vi "Utility Write To Register.vi"(7 "Unit Address (1)":u8=1, 8 "error in (no error)":errorcluster, 9 "Data (0)":i16, 10 "Register Address (0)":u16, 11 "VISA resource name":refnum<visa-resource-name>) -> (0 "error out":errorcluster {"code" format="%.0x"}, 3 "VISA resource name out":refnum<visa-resource-name>)   [LabVIEW 2014, in "Eurotherm 35xx Series.lvlib"]
doc: "This VI writes the value to the specified register of specified unit."
uses:
  <instrlib>/Eurotherm 35xx Series/Eurotherm 35xx Series.lvlib
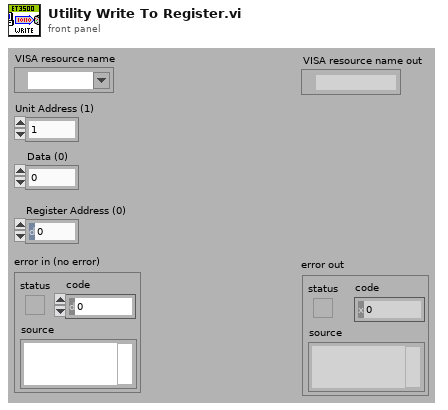
[diagram p1: front panel]
types:
  T1 = enum16{"By The Number of Bytes", "Copy Of the Sent Message"}
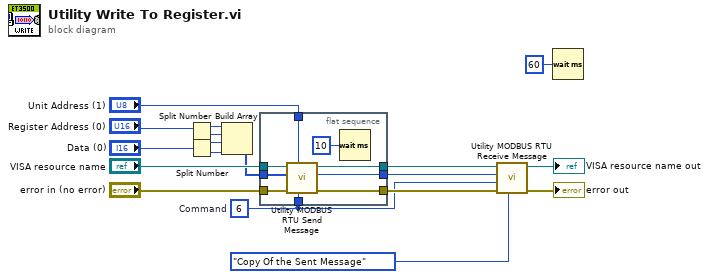
[diagram p0: block diagram]
diagram:
  w12 = u8 6  # Command
  n1 = Split Number(x="Register Address (0)") -> (hi(x)=w10:u8, lo(x)=w9:u8)
  n2 = Split Number(x="Data (0)") -> (hi(x)=w8:u8, lo(x)=w7:u8)
  n3 = Build Array(w10, w9, w8, w7) -> (w11:u8[])
  n4 = flat-sequence {
    tunnel: "VISA resource name" -> [w27]
    tunnel: "error in (no error)" -> [w26]
    tunnel: [w25] -> w14
    tunnel: [w24] -> w13
    tunnel: w12 -> [w23]
    tunnel: w11 -> [w22]
    tunnel: [w21] -> w6
    tunnel: "Unit Address (1)" -> [w20]
    frame #0 {
      n5 = call <instrlib>:"Utility MODBUS RTU Send Message.vi"("Command (0)"=w23, "Unit Address (1)"=w20, "error in (no error)"=w26, "Message (empty array)"=w22, "VISA resource name"=w27) -> ("error out"=w25:errorcluster, "Length Of Sent MSG"=w21:u8, "VISA resource name out"=w24:refnum<visa-resource-name>)  [unwired: 4 in]
      n6 = Wait (ms)(milliseconds to wait=u32 10) -> ()  [unwired: 1 out]
    }
  }
  n7 = call <instrlib>:"Utility MODBUS RTU Receive Message.vi"("Receive Message Type (0: By The Number Of Bytes)"=T1."Copy Of the Sent Message" ("Receive Message Type"), "error in (no error)"=w14, "Sent Command (0)"=w12, "Length Of Sent MSG (0)"=w6, "VISA resource name"=w13) -> ("error out"=→"error out":errorcluster, "VISA resource name out"=→"VISA resource name out":refnum<visa-resource-name>)  [unwired: 4 in, 1 out]
  n8 = Wait (ms)(milliseconds to wait=u32 60) -> ()  [unwired: 1 out]
